vi "Read Analog.vi"(0 "connection ID":refnum<k16>, 1 "address":u32, 2 "port":u16, 5 "Analog Number":u16, 9 "timeout ms (1000)":i32=1000, 11 "error in (no error)":errorcluster) -> (4 "connection ID out":refnum<k16>, 6 "received data":string, 8 "Analog Value":u16, 15 "error out":errorcluster)   [LabVIEW 2016, in "instr.lvlib"]
doc: "Reads analog value of given analog input."
uses:
  instr.lvlib
panel:
  out "Send String":string
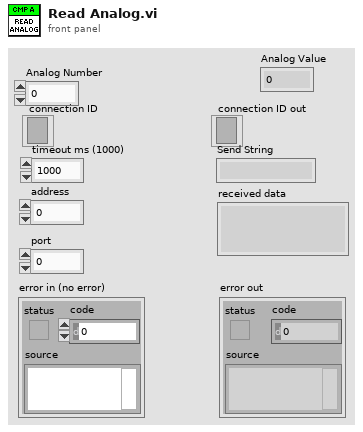
[diagram p1: front panel]
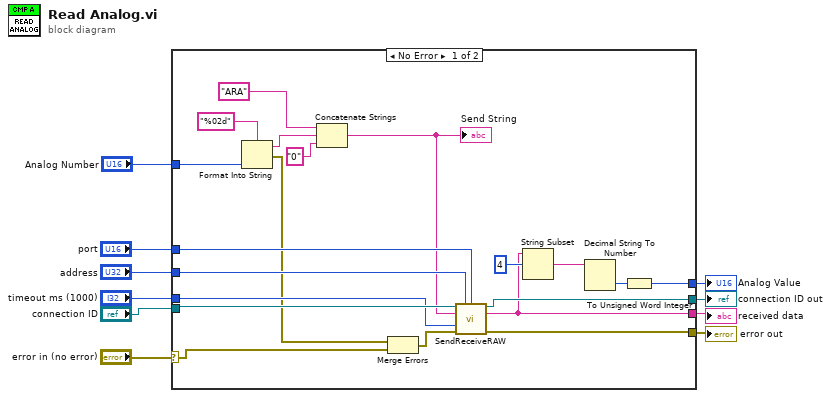
[diagram p0: block diagram]
diagram:
  n1 = case shown="No Error" "error in (no error)" {
    selector: "error in (no error)" -> [w17 w32]
    tunnel: [w30 w32] -> w10
    tunnel: "timeout ms (1000)" -> [w27 _]
    tunnel: "connection ID" -> [w28 w31]
    tunnel: [w29 w31] -> w6
    tunnel: "address" -> [w26 _]
    tunnel: "port" -> [w25 _]
    tunnel: [w23 _] -> w3
    tunnel: "Analog Number" -> [w18 _]
    tunnel: [w11 _] -> w1
    frame No Error {
      n2 = Format Into String(format string="%02d", w18) -> (resulting string=w19:string, error out=w14:errorcluster)  [unwired: 2 in]
      n3 = Concatenate Strings("ARA" ("data in"), w19, "0" ("string")) -> (w15:string)
      "Send String" <- w15
      n4 = Merge Errors(w14, w17) -> (w13:errorcluster)
      n5 = call "SendReceiveRAW.vi"("connection ID"=w28, "address"=w26, "port"=w25, "RAW data in"=w15, "timeout ms (1000)"=w27, "error in (no error)"=w13) -> ("connection ID out"=w29:refnum<k16>, "received data"=w23:string, "error out"=w30:errorcluster)  [unwired: 7 in]
      n6 = String Subset(string=w23, offset (0)=4 ("offset")) -> (substring=w12:string)  [unwired: 1 in]
      n7 = Decimal String To Number(string=w12) -> (number=w22:i32)  [unwired: 2 in, 1 out]
      n8 = To Unsigned Word Integer(number=w22) -> (unsigned 16bit integer=w11:u16)
    }
    frame Error {
    }
  }
  "error out" <- w10
  "received data" <- w3
  "connection ID out" <- w6
  "Analog Value" <- w1
